vi "Singulator Command Helper.vi"(7 "Description":string, 8 "Command Info In":T3, 11 "SubSystem Data":T1) -> (0 "Command Info Out":T3, 1 "Command Timing":cluster{"Start Time (ms)":u32, "Iterations":i32}, 3 "SubSystem Data":T1)   [LabVIEW 2019]
doc: "This VI shouldn't not be used directly, but is the core functionality of any given command. It is the primary communication path to the controller and stores the current command info."
uses:
  Singulator Setpoints.ctl
  Singulator Operations.ctl
  <vilib>/Rock Robotics/WPI/Framework/Command Status Info.ctl
  <vilib>/Rock Robotics/WPI/Framework/Completion Status.ctl
  <vilib>/Rock Robotics/WPI/Framework/Completion Notifier.ctl
  Singulator Published Globals.vi
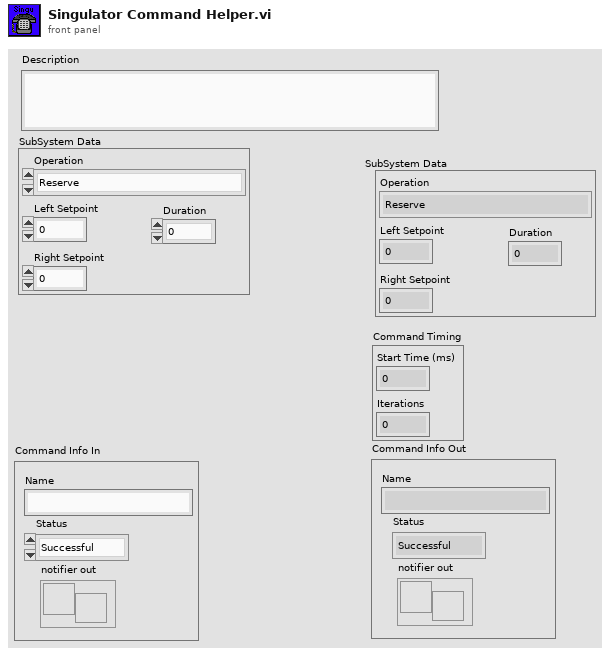
[diagram p1: front panel]
types:
  T1 = typedef "Singulator Setpoints.ctl" = cluster{"Operation":T2, "Left Setpoint":dbl, "Right Setpoint":dbl, "Duration":dbl}
  T2 = typedef "Singulator Operations.ctl" = enum16{"Reserve", "Singulate for time", "Read Current", "Immediate"}
  T3 = typedef "Command Status Info.ctl" = cluster{"Name":string, "Status":T4, "notifier out":T5}
  T4 = typedef "Completion Status.ctl" = enum16{"Successful", "Aborted", "Incomplete"}
  T5 = typedef "Completion Notifier.ctl" = refnum<notifier>
  T6 = cluster{"Current Command":T1, "Command Timing":cluster{"Start Time (ms)":u32, "Iterations":i32}, "Command Arguments":cluster{"Command Info":T3, "Description":string, "Default Command":T1, "queue out":refnum<queue>, "Subsystem Name":string}}
  T7 = cluster{"SubSystem Data":T1, "Command Info In":T3, string}
  T8 = cluster{"Command Info":T3, "Description":string, "Default Command":T1, "queue out":refnum<queue>, "Subsystem Name":string}
  T9 = cluster{"SubSystem Data":T1, "Command Info In":T3, "Description":string}
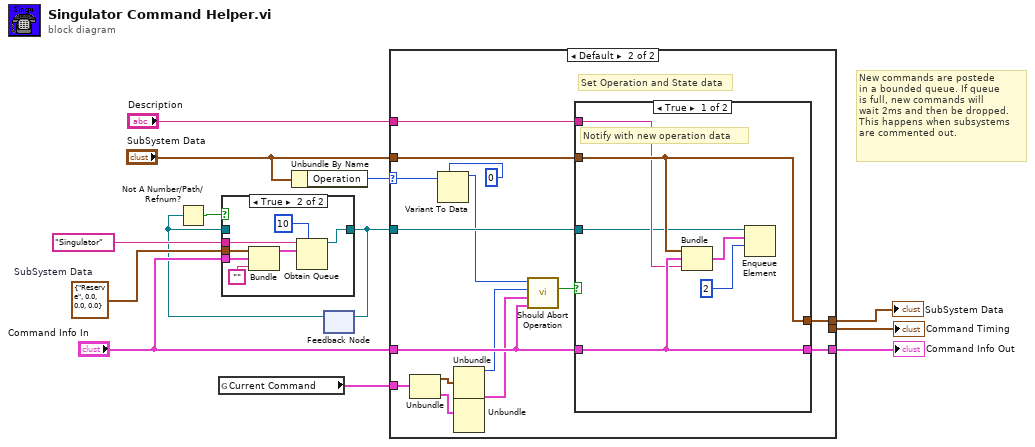
[diagram p0: block diagram]
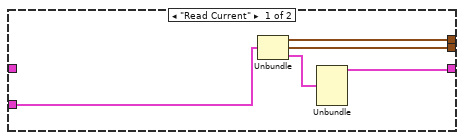
[diagram p3: hidden frame]
diagram:
  w8 = T1 {"Operation"=enum."Reserve", "Left Setpoint"=0.0, "Right Setpoint"=0.0, "Duration"=0.0}  # SubSystem Data
  # "New commands are postede\nin a bounded queue. If queue\nis full, new commands will\nwait 2ms and then be dropped.\nThis happens when subsystems\nare commented out."
  n1 = global read "Singulator Published Globals.vi" "Current Command"() -> (w2:T6)
  n2 = Unbundle By Name("SubSystem Data") -> ("Operation"=w1:T2)
  n3 = feedback #1() -> (w5:refnum<queue>)  [unwired: 1 in]
  n4 = Not A Number/Path/Refnum?(number/path/refnum=w5) -> (NaN/Path/Refnum?=w6:bool)
  n5 = case shown="True" w6 {
    tunnel: "Singulator" -> [_ w18]
    tunnel: [w14 w16] -> w11
    tunnel: w8 -> [_ w21]
    tunnel: "Command Info In" -> [_ w20]
    tunnel: w5 -> [w14 _]
    frame False {
    }
    frame True {
      n6 = Bundle("SubSystem Data"=w21, "Command Info In"=w20, "") -> (w17:T7)  [unwired: 1 in]
      n7 = Obtain Queue(max queue size (-1, unlimited)=10, name (unnamed)=w18, element data type=w17) -> (queue out=w16:refnum<queue>)  [unwired: 2 in, 2 out]
    }
  }
  n8 = feedback-in #1(w11) -> ()
  n9 = case shown="Default" w1 {
    selector: w1 -> [_ w29]
    tunnel: [w25 w38] -> w7
    tunnel: w11 -> [_ w40]
    tunnel: "SubSystem Data" -> [_ w41]
    tunnel: [w24 w39] -> w10
    tunnel: "Command Info In" -> [_ w36]
    tunnel: "Description" -> [_ w35]
    tunnel: [w23 _] -> w3
    tunnel: w2 -> [w22 w34]
    frame "Read Current" {
      n10 = Unbundle(w22) -> ("Current Command"=w25:T1, "Command Timing"=w23:cluster{"Start Time (ms)":u32, "Iterations":i32}, "Command Arguments"=w26:T8)
      n11 = Unbundle(w26) -> ("Command Info"=w24:T3)  [unwired: 4 out]
    }
    frame Default {
      # "Set Operation and State data"
      n12 = Unbundle(w34) -> ("Current Command"=w33:T1, "Command Arguments"=w31:T8)  [unwired: 1 out]
      n13 = Variant To Data(type=0, Variant=w29) -> (data=w27:i32)  [unwired: 1 in, 1 out]
      n14 = Unbundle(w33) -> ("Operation"=w32:T2)  [unwired: 3 out]
      n15 = Unbundle(w31) -> ("Command Info"=w30:T3)  [unwired: 4 out]
      n16 = call <vilib>:"Should Abort Operation.vi"("New Command Info"=w36, "Command Info"=w30, "Current Operation"=w32, "New Operation"=w27) -> ("Execute"=w37:bool)  [unwired: 7 in]
      n17 = case shown="True" w37 {
        tunnel: [w47 _] -> w38
        tunnel: w41 -> [w47 _]
        tunnel: w40 -> [w44 _]
        tunnel: [w46 w48] -> w39
        tunnel: w36 -> [w46 w48]
        tunnel: w35 -> [w45 _]
        frame True {
          # "Notify with new operation data"
          n18 = Bundle("SubSystem Data"=w47, "Command Info In"=w46, "Description"=w45) -> (w43:T9)  [unwired: 1 in]
          n19 = Enqueue Element(queue=w44, element=w43, timeout in ms (-1)=2 ("max queue size (-1, unlimited)")) -> ()  [unwired: 1 in, 3 out]
        }
        frame False {
          # "This operation will not be\nexecuted. Upstream command\nwas aborted."
        }
      }
    }
  }
  "Command Info Out" <- w10
  "SubSystem Data" <- w7
  "Command Timing" <- w3
